vi "GenerateUntriggeredStimulus.vi"(8 "error in (no error)":errorcluster, 11 "StimulusObject in":refnum<class "StimulusObject.lvclass">) -> (0 "error out":errorcluster, 2 "UntriggeredStimulusOut":sgl[][](array[numeric]), 3 "StimulusObject out":refnum<class "StimulusObject.lvclass">)   [LabVIEW 2019, in "StimulusObject.lvclass"]
uses:
  StimulusObject.lvclass
  ParametersGlobal.vi
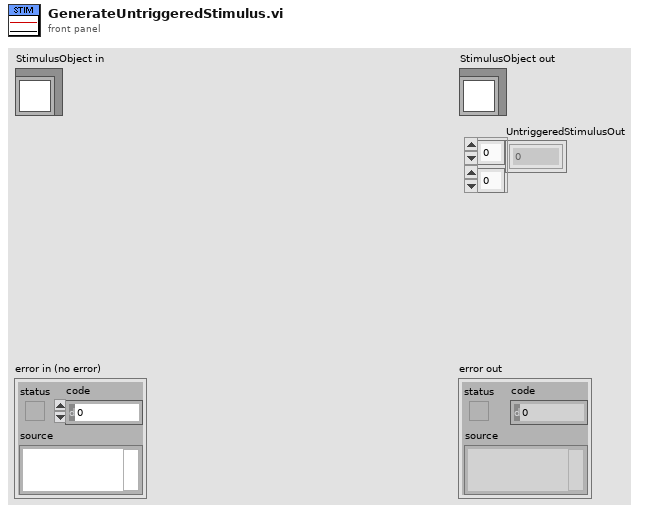
[diagram p1: front panel]
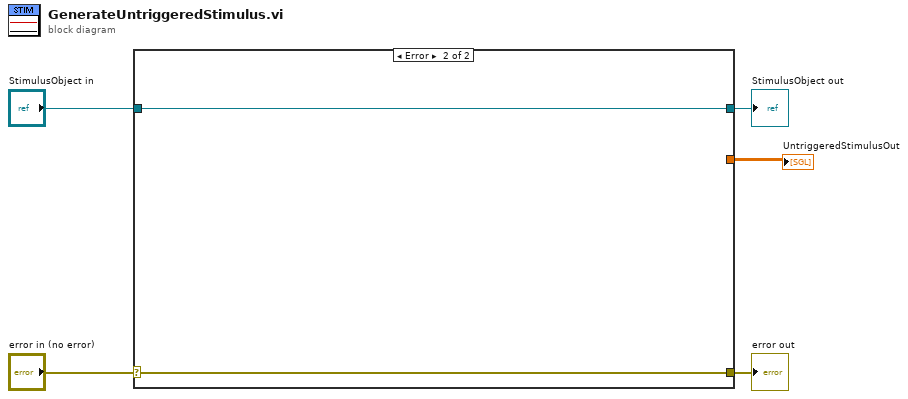
[diagram p0: block diagram]
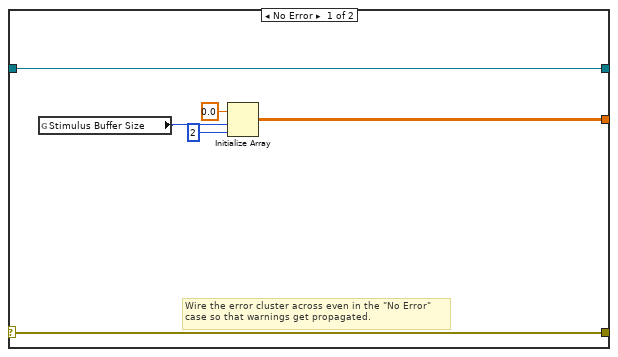
[diagram p2: hidden frame]
diagram:
  n1 = case shown="Error" "error in (no error)" {
    selector: "error in (no error)" -> [w11 w13]
    tunnel: [w11 w13] -> w4
    tunnel: [w8 w12] -> w2
    tunnel: "StimulusObject in" -> [w8 w12]
    tunnel: [w6 _] -> w1
    frame No Error {
      # "Wire the error cluster across even in the \"No Error\"\ncase so that warnings get propagated."
      n2 = global read "ParametersGlobal.vi" "Stimulus Buffer Size"() -> (w7:i32)
      n3 = Initialize Array(sgl 0.0 ("element"), w7, 2 ("dimension size")) -> (w6:sgl[][])
    }
    frame Error {
    }
  }
  "error out" <- w4
  "StimulusObject out" <- w2
  "UntriggeredStimulusOut" <- w1
